vi "CH_LM Calibration Hardware Override.vi"(0 "Meter Index":i32, 2 "Hardware Calibration":T1={"Pyro DAC Attenuator"=0, "Pyro Input Attenuator"=1, "Q Control"=0, "S Control"=0, "G Control"=0, "P Control"=0}, 5 "error in (no error)":errorcluster, 7 "Timeout / ms (3000)":i32=3000, 8 "Action (query)":bool, 9 "Lock Timeout / ms (1000)":i32=1000) -> (11 "Lock timed out":bool, 14 "Meter Index":i32, 16 "Hardware Calibration":T1={"Pyro DAC Attenuator"=0, "Pyro Input Attenuator"=1, "Q Control"=0, "S Control"=0, "G Control"=0, "P Control"=0}, 19 "error out":errorcluster)   [LabVIEW 2012, in "CH_LM.lvlib"]
doc: "This command overrides/queries the current values for the following analog circuit control points:\n\n- Pyro DAC attenuator\n- Pyro input attenuator\n- T control\n- S control\n- G control\n- P control\n\n<B>Attention:</B> This command will result in the meter entering a calibration state under which calibration is possible but normal meter operation is not possible. A power off/on cycle will place the meter into a normal operational mode."
uses:
  CH_LM.lvlib
  CH_LM Calibration Hardware Override.ctl
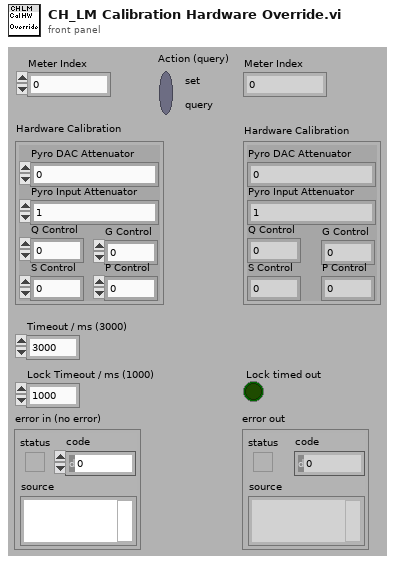
[diagram p1: front panel]
types:
  T1 = typedef "CH_LM.lvlib/CH_LM Calibration Hardware Override.ctl" = cluster{"Pyro DAC Attenuator":i32, "Pyro Input Attenuator":i32, "Q Control":i32, "S Control":i32, "G Control":i32, "P Control":i32}
  T2 = cluster{"Pyro DAC Attenuator":bool, "Pyro Input Attenuator":bool, "Q Control":bool, "S Control":bool, "G Control":bool, "P Control":bool}
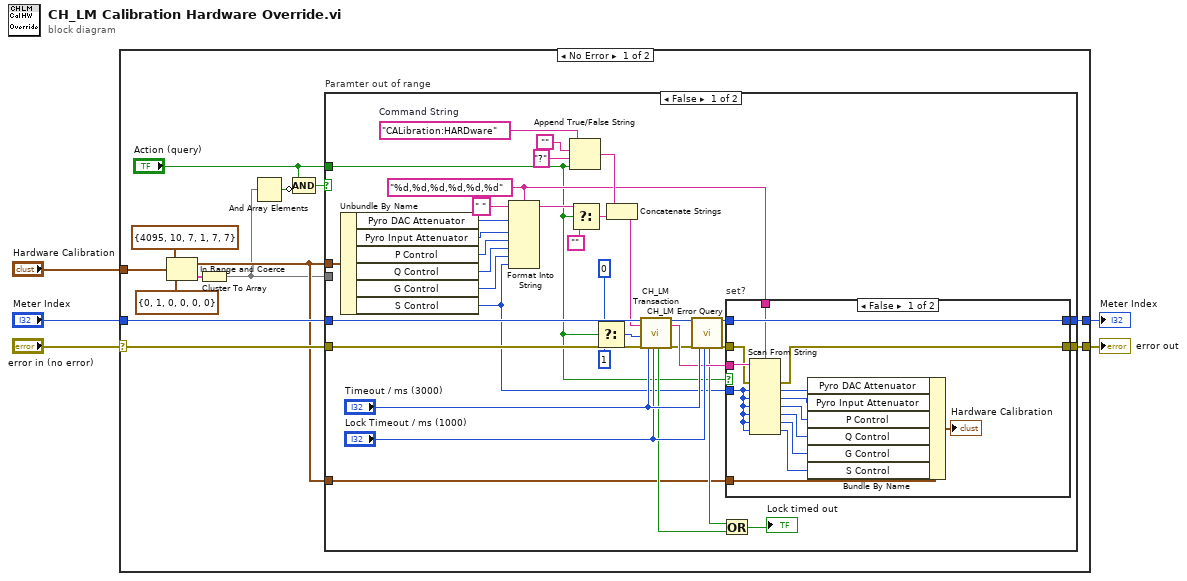
[diagram p0: block diagram]
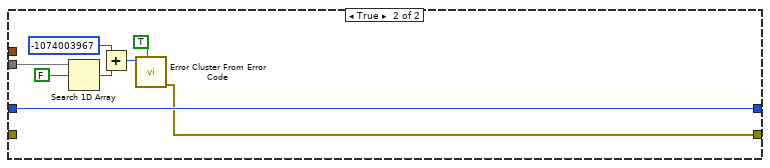
[diagram p3: hidden frame]
diagram:
  n1 = case shown="No Error" "error in (no error)" {
    selector: "error in (no error)" -> [w18 w80]
    tunnel: [w16 w80] -> w5
    tunnel: "Meter Index" -> [w17 w79]
    tunnel: [w15 w79] -> w2
    tunnel: "Hardware Calibration" -> [w10 _]
    frame No Error {
      n2 = In Range and Coerce(upper limit=T1 {"Pyro DAC Attenuator"=4095, "Pyro Input Attenuator"=10, "Q Control"=7, "S Control"=1, "G Control"=7, "P Control"=7}, x=w10, lower limit=T1 {"Pyro DAC Attenuator"=0, "Pyro Input Attenuator"=1, "Q Control"=0, "S Control"=0, "G Control"=0, "P Control"=0}) -> (coerced(x)=w9:T1, In Range?=w11:T2)
      n3 = Cluster To Array(cluster=w11) -> (array=w7:bool[])
      n4 = And Array Elements(Boolean array=w7) -> (logical AND=w8:bool)
      n5 = Compound Arithmetic op=AND("Action (query)", invert w8) -> (w14:bool)
      n6 = case "Paramter out of range" shown="False" w14 {
        tunnel: w18 -> [w54 _]
        tunnel: w17 -> [w53 w78]
        tunnel: [w52 w71] -> w16
        tunnel: [w51 w78] -> w15
        tunnel: w9 -> [w23 _]
        tunnel: "Action (query)" -> [w20 _]
        tunnel: w9 -> [w19 _]
        tunnel: w7 -> [_ w76]
        frame False {
          w25 = "%d,%d,%d,%d,%d,%d" ("format string")
          w48 = "CALibration:HARDware"  # Command String
          n7 = Unbundle By Name(w23) -> ("Pyro DAC Attenuator"=w29:i32, "Pyro Input Attenuator"=w28:i32, "P Control"=w27:i32, "Q Control"=w24:i32, "G Control"=w22:i32, "S Control"=w21:i32)
          n8 = Format Into String(format string=w25, initial string=" " ("string"), w29, w28, w27, w24, w22, w21) -> (resulting string=w26:string)  [unwired: 1 in, 1 out]
          n9 = Append True/False String(1:w20, 2:"?" ("true string"), 3:"", 4:w48) -> (0:w31:string)
          n10 = Select(t=w26, s=w20, f="") -> (s? t:f=w44:string)
          n11 = Select(t=0, s=w20, f=1 ("NofStrings (-1:all)")) -> (s? t:f=w41:i32)
          n12 = Concatenate Strings(w31, w44) -> (w32:string)
          n13 = call "CH_LM Transaction.vi"("Meter Index"=w53, "Command String"=w32, "NofStrings (-1:all)"=w41, "error in (no error)"=w54, "Timeout / ms (3000)"="Timeout / ms (3000)", "Lock Timeout / ms (1000)"="Lock Timeout / ms (1000)") -> ("Lock timed out"=w34:bool, "Meter Index"=w39:i32, "Response"=w47:string, "error out"=w37:errorcluster)  [unwired: 10 out]
          n14 = call "CH_LM Error Query.vi"("Meter Index"=w39, "error in (no error)"=w37, "Timeout / ms (3000)"="Timeout / ms (3000)", "Lock Timeout / ms (1000)"="Lock Timeout / ms (1000)") -> ("Lock timed out"=w35:bool, "Meter Index"=w38:i32, "error out"=w36:errorcluster)  [unwired: 13 out]
          n15 = Or(x=w35, y=w34) -> (x .or. y?=→"Lock timed out":bool)
          n16 = case "set?" shown="False" w20 {
            tunnel: w47 -> [w67 _]
            tunnel: w36 -> [w65 w69]
            tunnel: [w64 w69] -> w52
            tunnel: w38 -> [w68 w70]
            tunnel: [w68 w70] -> w51
            tunnel: w25 -> [w66 _]
            tunnel: w21 -> [w58 _]
            tunnel: w19 -> [w63 _]
            frame False {
              n17 = Scan From String(format string=w66, input string=w67, error in=w65, default 1=w58, default 2=w58, default 3=w58, default 4=w58, default 5=w58, default 6=w58) -> (error out=w64:errorcluster, output 1=w62:i32, output 2=w61:i32, output 3=w60:i32, output 4=w59:i32, output 5=w57:i32, output 6=w56:i32)  [unwired: 1 in, 2 out]
              n18 = Bundle By Name(cluster=w63, "Pyro DAC Attenuator"=w62, "Pyro Input Attenuator"=w61, "P Control"=w60, "Q Control"=w59, "G Control"=w57, "S Control"=w56) -> (→"Hardware Calibration":T1)
            }
            frame True {
            }
          }
        }
        frame True {
          n19 = Search 1D Array(1D array=w76, element=FALSE) -> (index of element=w73:i32)  [unwired: 1 out]
          n20 = Add(x=-1074003967 ("error code (0)"), y=w73) -> (x+y=w72:i32)
          n21 = call <vilib>:"Error Cluster From Error Code.vi"("show call chain? (False)"=TRUE, "error code (0)"=w72) -> ("error out"=w71:errorcluster)  [unwired: 1 in, 6 out]
        }
      }
    }
    frame Error {
    }
  }
  "error out" <- w5
  "Meter Index" <- w2
